vi "SimpleGetPeaks.vi"(8 "Error In":errorcluster, 11 "Address":string="10.0.0.55") -> (0 "Error Out":errorcluster, 3 "Peaks Data":T1 {"Peaks Wvls, nm"."Peak Wvls, nm" format="%#_8g"})   [LabVIEW 2016]
doc: "This example VI demonstrates the use of the #GetPeaks command to retrieve peaks data from Hyperion instruments."
uses:
  h.Library/ACQ/CTL/h.ACQ.PeaksData.ctl
  h.Library/ACQ/CTL/h.ACQ.PeaksWvl.ctl
  h.Library.lvlib
panel:
  # "Hyperion Simple #GetPeaks Example"
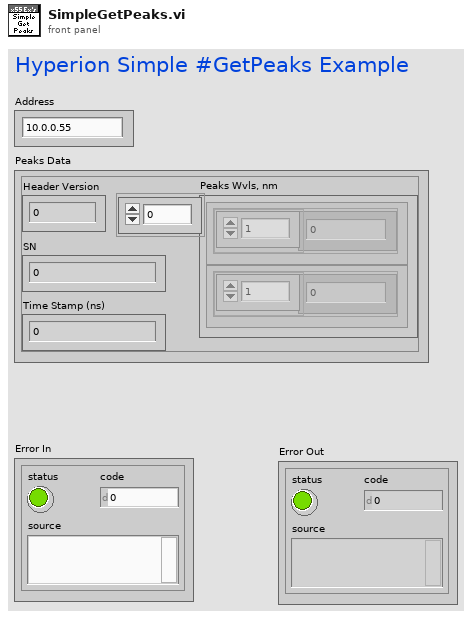
[diagram p1: front panel]
types:
  T1 = typedef "h.Library.lvlib/h.ACQ.PeaksData.ctl" = cluster{"SN":u64, "Time Stamp (ns)":u64, "Header Version":u16, "Peaks Wvls, nm":T2[]}
  T2 = typedef "h.Library.lvlib/h.ACQ.PeaksWvl.ctl" = cluster{"Peak Wvls, nm":dbl[]}
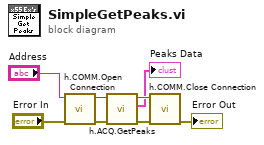
[diagram p0: block diagram]
diagram:
  n1 = call "h.COMM.Open Connection.vi"("error in"="Error In", "Address"="Address") -> ("error out"=w5:errorcluster, "Connection ID"=w7:refnum<k5>)  [unwired: 8 in]
  n2 = call "h.ACQ.GetPeaks.vi"("error in"=w5, "Connection ID In"=w7) -> ("error out"=w4:errorcluster, "Peaks Data"=→"Peaks Data":T1, "Connection ID Out"=w6:refnum<k5>)  [unwired: 7 in]
  n3 = call "h.COMM.Close Connection.vi"("error in"=w4, "Connection ID"=w6) -> ("error out"=→"Error Out":errorcluster)  [unwired: 9 in]
